vi "Load Info.vi"(8 "error in":errorcluster, 11 "filename":path) -> (0 "error out":errorcluster, 3 "info data":string)   [LabVIEW 2020, in "infolib.lvlib"]
doc: "Reads whole info file. If filename not found, extension '.info' is added. If still no file found, error is generated."
uses:
  infolib.lvlib
  <vilib>/Utility/error.llb/Error Cluster From Error Code.vi
  <vilib>/ErrorRing/Error Ring.xnode
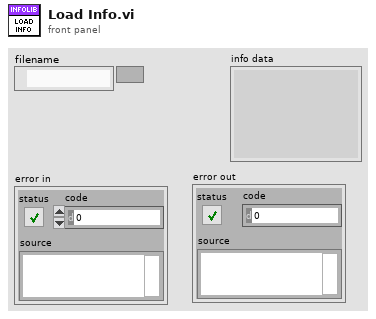
[diagram p1: front panel]
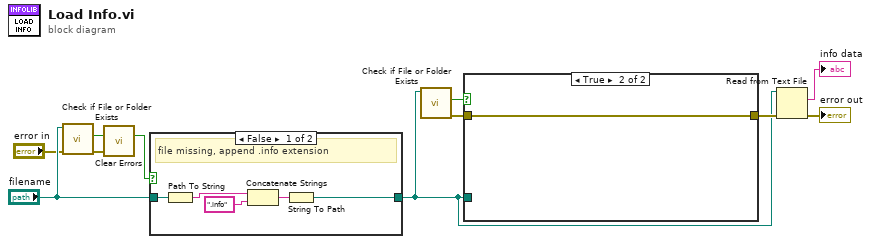
[diagram p0: block diagram]
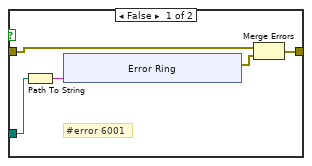
[diagram p3: hidden frame]
diagram:
  n1 = call <vilib>:"Check if File or Folder Exists.vi"("error in (no error)"="error in", "path"="filename") -> ("error out"=w1:errorcluster, "file or folder exists?"=w3:bool)  [unwired: 7 in, 1 out]
  n2 = call <vilib>:"Clear Errors.vi"("error in (no error)"=w1) -> ()  [unwired: 5 in, 2 out]
  n3 = case shown="False" w3 {
    tunnel: [w15 w16] -> w8
    tunnel: "filename" -> [w14 w16]
    frame False {
      # "file missing, append .info extension"
      n4 = Path To String(path=w14) -> (string=w12:string)
      n5 = Concatenate Strings(w12, ".info" ("y")) -> (w11:string)
      n6 = String To Path(string=w11) -> (path=w15:path)
    }
    frame True {
      # "file exist, do not append .info extension"
    }
  }
  n7 = call <vilib>:"Check if File or Folder Exists.vi"("path"=w8) -> ("error out"=w6:errorcluster, "file or folder exists?"=w7:bool)  [unwired: 8 in, 1 out]
  n8 = case shown="True" w7 {
    tunnel: w6 -> [w21 w29]
    tunnel: [w19 w29] -> w9
    tunnel: w8 -> [w17 _]
    frame False {
      # "#error 6001"
      n9 = Path To String(path=w17) -> (string=w18:string)
      n10 = xnode "Error Ring"("parameter 0"=w18) -> ("error out"=w20:errorcluster)
      n11 = Merge Errors(w21, w20) -> (w19:errorcluster)
    }
    frame True {
    }
  }
  n12 = Read from Text File(file (use dialog)=w8, error in=w9) -> (text=→"info data":string, error out=→"error out":errorcluster)  [unwired: 2 in, 2 out]
